vi "UserAddedRow Event Callback.vi"(4 "DataGridView in":refnum<class "DataGridView.lvclass">, 5 "Event Data":cluster{"sender":refnum<k24>, "e":refnum<k24>}, 6 "Control Ref":refnum<k24>, 7 "Event Common Data":T1) -> ()   [LabVIEW 2014, in "DataGrid.lvlib" / "DataGridView.lvclass"]
uses:
  DataGridView/DataGridView.lvclass
  System.Windows.Forms
  Controls/EventsList.ctl
  UserAddedRow/UserAddedRow.lvclass
  UserAddedRow/UserAddedRow.lvclass/UserAddedRow.ctl
  UserAddedRow/Write Row.vi
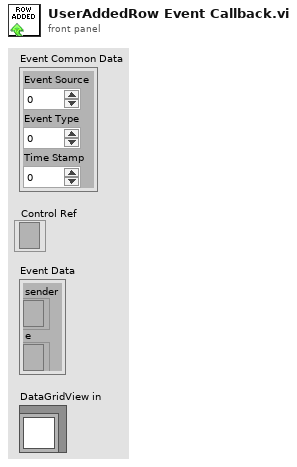
[diagram p1: front panel]
types:
  T1 = cluster{"Event Source":i32, "Event Type":u32, "Time Stamp":u32}
  T2 = typedef "DataGrid.lvlib/DataGridView.lvclass/EventsList.ctl" = enum16{"CellClicked", "CellValueChanged", "KeyDown", "DataError", "UserAddedRow", "UserDeletedRow"}
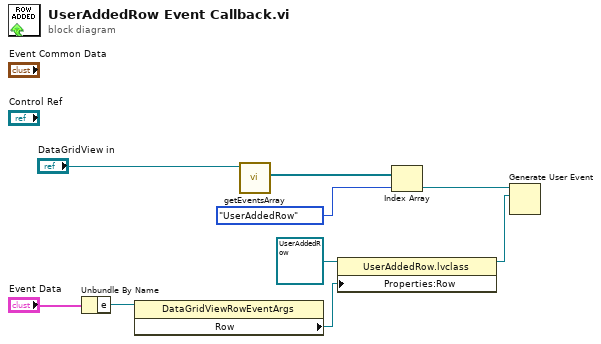
[diagram p0: block diagram]
diagram:
  n1 = Unbundle By Name("Event Data") -> ("e"=w4:refnum<k24>)
  n2 = property class="DataGridViewRowEventArgs"(reference=w4) -> ("Row"=w2:refnum<k24>)  [unwired: 1 in, 2 out]
  n3 = call "getEventsArray.vi"("DataGridView in"="DataGridView in") -> ("userEvents"=w8:refnum<user-event>[])  [unwired: 8 in, 2 out]
  n4 = property class="UserAddedRow.lvclass"(reference=refnum<class "UserAddedRow.lvclass"> refnum ("DataGrid.lvlib:UserAddedRow.lvclass"), "Properties:Row"=w2) -> (reference out=w1:refnum<class "UserAddedRow.lvclass">)  [unwired: 1 in, 1 out]
  n5 = Index Array(array=w8, index=EventsList."UserAddedRow") -> (element=w7:refnum<user-event>)
  n6 = Generate User Event(user event=w7, event data cluster=w1) -> ()  [unwired: 2 in, 2 out]
